vi "Configure Keylock.vi"(7 "Unit Address (1)":u8=1, 8 "error in (no error)":errorcluster, 10 "Enable Keylock (False: Unlock)":bool, 11 "VISA resource name":refnum<visa-resource-name>) -> (0 "error out":errorcluster, 3 "VISA resource name out":refnum<visa-resource-name>)   [LabVIEW 2014, in "Eurotherm 35xx Series.lvlib"]
doc: "This VI locks or unlocks instrument keys."
uses:
  <instrlib>/Eurotherm 35xx Series/Eurotherm 35xx Series.lvlib
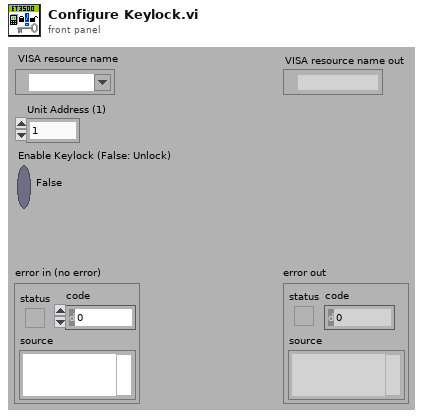
[diagram p1: front panel]
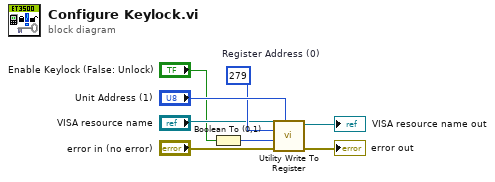
[diagram p0: block diagram]
diagram:
  w5 = u16 279  # Register Address (0)
  n1 = Boolean To (0,1)(Boolean="Enable Keylock (False: Unlock)") -> (0, 1=w2:i16)
  n2 = call <instrlib>:"Utility Write To Register.vi"("Unit Address (1)"="Unit Address (1)", "error in (no error)"="error in (no error)", "Data (0)"=w2, "Register Address (0)"=w5, "VISA resource name"="VISA resource name") -> ("error out"=→"error out":errorcluster, "VISA resource name out"=→"VISA resource name out":refnum<visa-resource-name>)  [unwired: 5 in]
